vi "Data Parser.vi"(10 "Incoming Data in":u8[](array[numeric])) -> (0 "Clear":i16 format="%x   %.0f", 1 "Blue":i16 format="%x   %.0f", 2 "Green":i16 format="%x   %.0f", 3 "RED":i16 format="%x", 4 "Gain Value":i32, 5 "A-TIME-MS":dbl, 6 "A-GAIN":u8, 7 "A-TIME":u8 format="%.0f  %x")   [LabVIEW 2014, in "AMS TS3472 Light Sensor.lvlib" / "AMS TCS3472.lvclass"]
uses:
  AMS TCS3472.lvclass
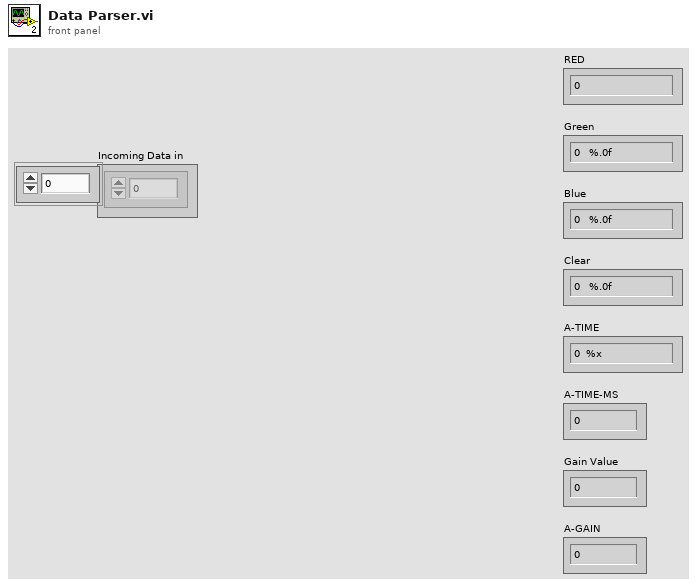
[diagram p1: front panel]
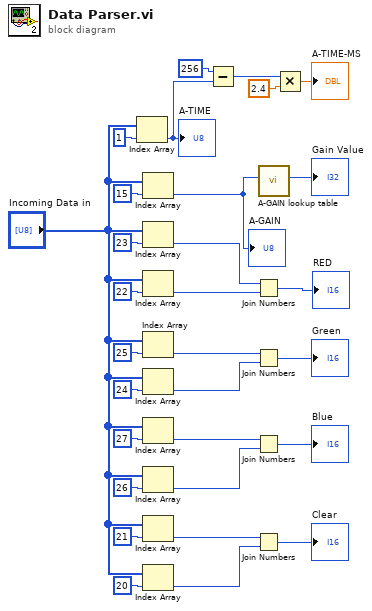
[diagram p0: block diagram]
diagram:
  n1 = Index Array(array="Incoming Data in", index=1) -> (element=w25:u8)
  "A-TIME" <- w25
  n2 = Index Array(array="Incoming Data in", index=15) -> (element=w28:u8)
  "A-GAIN" <- w28
  n3 = Index Array(array="Incoming Data in", index=23) -> (element=w15:u8)
  n4 = Index Array(array="Incoming Data in", index=22) -> (element=w14:u8)
  n5 = Index Array(array="Incoming Data in", index=25) -> (element=w13:u8)
  n6 = Index Array(array="Incoming Data in", index=24) -> (element=w12:u8)
  n7 = Index Array(array="Incoming Data in", index=27) -> (element=w10:u8)
  n8 = Index Array(array="Incoming Data in", index=26) -> (element=w11:u8)
  n9 = Index Array(array="Incoming Data in", index=21) -> (element=w17:u8)
  n10 = Index Array(array="Incoming Data in", index=20) -> (element=w16:u8)
  n11 = Subtract(x=u16 256, y=w25) -> (x-y=w26:u16)
  n12 = Join Numbers(hi=w15, lo=w14) -> ((hi.lo)=→"RED":u16)
  n13 = Join Numbers(hi=w13, lo=w12) -> ((hi.lo)=→"Green":u16)
  n14 = Join Numbers(hi=w10, lo=w11) -> ((hi.lo)=→"Blue":u16)
  n15 = Join Numbers(hi=w17, lo=w16) -> ((hi.lo)=→"Clear":u16)
  n16 = call "A-GAIN lookup table.vi"("Enum"=w28) -> ("Gain Value"=→"Gain Value":i32)  [unwired: 10 in]
  n17 = Multiply(x=w26, y=2.4) -> (x*y=→"A-TIME-MS":dbl)
